vi "Growable Widget.vi"(8 "Error In":errorcluster, 10 "Widget Builder":refnum<class "Abstract Widget Builder.lvclass">) -> (0 "Error Out":errorcluster, 3 "New Growable Widget":refnum<class "Growable Widget.lvclass">)   [LabVIEW 2014, in "Dynamic GUI Composition and Management.lvlib" / "Growable Widget.lvclass"]
doc: "Copyright (c) 2016 Sze Howe Koh\nThis code is licensed under the MIT license"
uses:
  Growable Widget.lvclass
  Widget Builders/Abstract Widget Builder/Abstract Widget Builder.lvclass
  src/LabVIEW/Qt Widgets/QBoxLayout/Direction.ctl
  src/LabVIEW/Qt Widgets/QFrame/Shadow.ctl
  src/LabVIEW/Qt Widgets/QFrame/Shape.ctl
  Growable Widget.lvclass/Growable Widget.ctl
  src/LabVIEW/Qt Widgets/QFrame/setFrameShadow.vi
  src/LabVIEW/Qt Widgets/QFrame/setFrameShape.vi
  src/LabVIEW/LQ Core/LQCoreEngine/_Polymorphic Instances/Connect_CallbackIn_Void.vi
  src/LabVIEW/Qt Widgets/QComboBox/QComboBox.lvclass
  src/LabVIEW/Qt Widgets/QPushButton/QPushButton.lvclass
  src/LabVIEW/Qt Widgets/QBoxLayout/QBoxLayout.lvclass
  src/LabVIEW/Qt Widgets/QWidget/QWidget.lvclass
  src/LabVIEW/LQ Core/LQCoreEngine/LQCoreEngine.lvclass
  src/LabVIEW/Qt Widgets/QLineEdit/QLineEdit.lvclass
  src/LabVIEW/Qt Widgets/QFrame/QFrame.lvclass
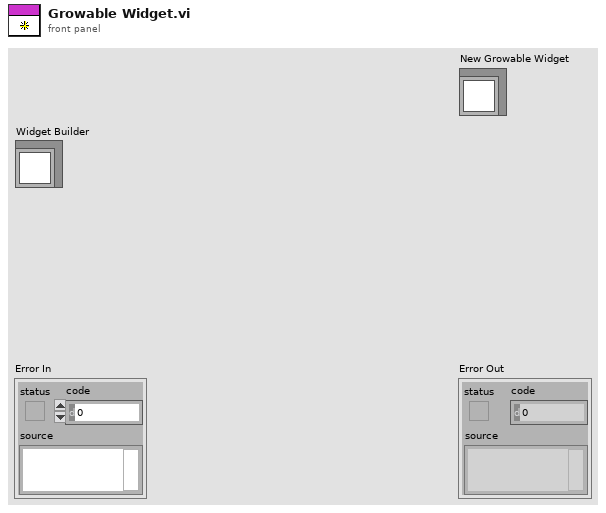
[diagram p1: front panel]
types:
  T1 = typedef "QFrame.lvclass/Shape.ctl" = i32
  T2 = typedef "QFrame.lvclass/Shadow.ctl" = i32
  T3 = typedef "QBoxLayout.lvclass/Direction.ctl" = i32
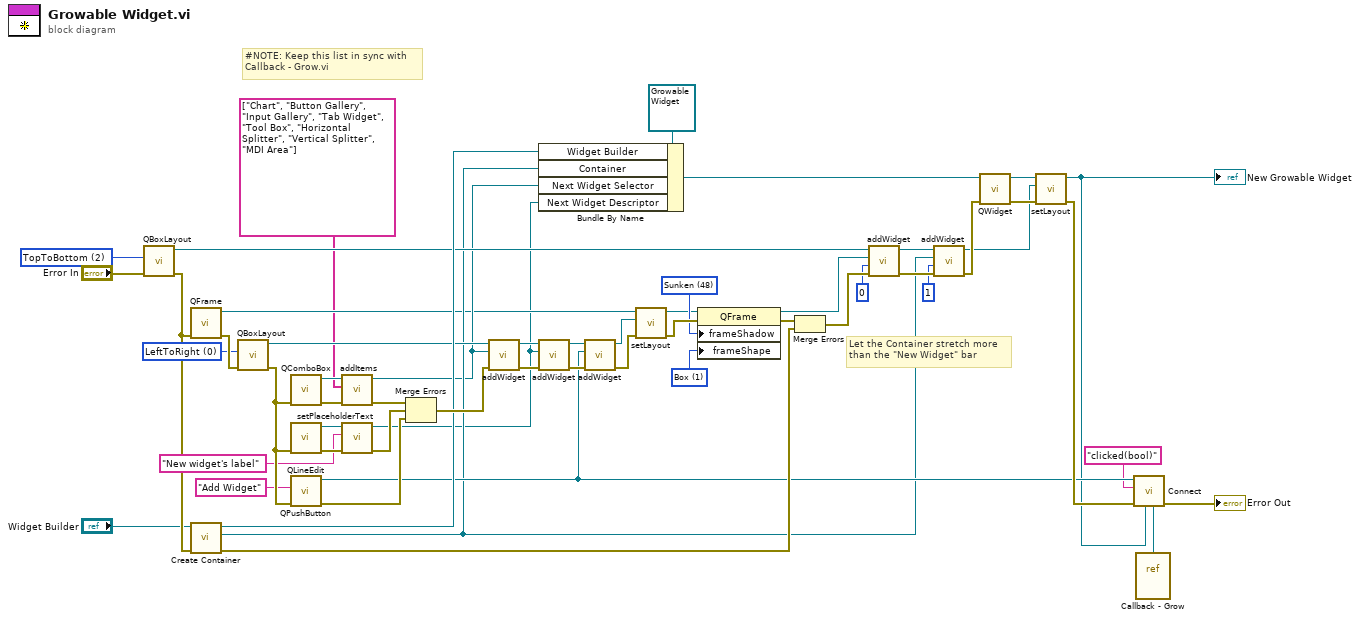
[diagram p0: block diagram]
diagram:
  w18 = T1 1 items=["NoFrame", "Box", "Panel", "HLine", "VLine", "StyledPanel"] ("frameShape")
  w19 = T2 48 items=["Plain"=16, "Raised"=32, "Sunken"=48] ("frameShadow")
  w36 = T3 2 items=["LeftToRight", "RightToLeft", "TopToBottom", "BottomToTop"] ("direction")
  w37 = T3 0 items=["LeftToRight", "RightToLeft", "TopToBottom", "BottomToTop"] ("direction")
  # "Let the Container stretch more\nthan the \"New Widget\" bar"
  # "#NOTE: Keep this list in sync with\nCallback - Grow.vi"
  n1 = call "QBoxLayout.vi"("Error In"="Error In", "direction"=w36) -> ("Error Out"=w54:errorcluster, "New QBoxLayout"=w32:refnum<class "QBoxLayout.lvclass">)  [unwired: 8 in]
  n2 = call "QFrame.vi"("Error In"=w54) -> ("Error Out"=w40:errorcluster, "New QFrame"=w20:refnum<class "QFrame.lvclass">)  [unwired: 9 in]
  n3 = call-dynamic "Create Container.vi"("Error In"=w54, "Abstract Widget Builder in"="Widget Builder") -> ("Error Out"=w53:errorcluster, "Container"=w24:refnum<class "QWidget.lvclass">, "Abstract Widget Builder out"=w48:refnum<class "Abstract Widget Builder.lvclass">)  [unwired: 7 in]
  n4 = call "QBoxLayout.vi"("Error In"=w40, "direction"=w37) -> ("Error Out"=w44:errorcluster, "New QBoxLayout"=w39:refnum<class "QBoxLayout.lvclass">)  [unwired: 8 in]
  n5 = call "QComboBox.vi"("Error In"=w44) -> ("Error Out"=w13:errorcluster, "New QComboBox"=w41:refnum<class "QComboBox.lvclass">)  [unwired: 9 in]
  n6 = call "QLineEdit.vi"("Error In"=w44) -> ("Error Out"=w4:errorcluster, "New QLineEdit"=w6:refnum<class "QLineEdit.lvclass">)  [unwired: 9 in]
  n7 = call "QPushButton.vi"("Error In"=w44, "text"="Add Widget") -> ("Error Out"=w43:errorcluster, "New QPushButton"=w26:refnum<class "QPushButton.lvclass">)  [unwired: 8 in]
  n8 = call "addItems.vi"("Error In"=w13, "texts"=string[] ["Chart", "Button Gallery", "Input Gallery", "Tab Widget", "Tool Box", "Horizontal Splitter", "Vertical Splitter", "MDI Area"], "QComboBox In"=w41) -> ("Error Out"=w12:errorcluster, "QComboBox Out"=w23:refnum<class "QComboBox.lvclass">)  [unwired: 7 in]
  n9 = call "setPlaceholderText.vi"("Error In"=w4, "text"="New widget's label", "QLineEdit In"=w6) -> ("Error Out"=w47:errorcluster, "QLineEdit Out"=w5:refnum<class "QLineEdit.lvclass">)  [unwired: 7 in]
  n10 = Merge Errors(w12, w47, w43) -> (w49:errorcluster)
  n11 = call "addWidget.vi"("Error In"=w49, "widget"=w23, "QBoxLayout In"=w39) -> ("Error Out"=w11:errorcluster, "QBoxLayout Out"=w22:refnum<class "QBoxLayout.lvclass">)  [unwired: 7 in]
  n12 = Bundle By Name(cluster=refnum<class "Growable Widget.lvclass"> refnum ("Growable Widget"), "Widget Builder"=w48, "Container"=w24, "Next Widget Selector"=w23, "Next Widget Descriptor"=w5) -> (w33:refnum<class "Growable Widget.lvclass">)
  n13 = call "addWidget.vi"("Error In"=w11, "widget"=w5, "QBoxLayout In"=w22) -> ("Error Out"=w46:errorcluster, "QBoxLayout Out"=w21:refnum<class "QBoxLayout.lvclass">)  [unwired: 7 in]
  n14 = call "addWidget.vi"("Error In"=w46, "widget"=w26, "QBoxLayout In"=w21) -> ("Error Out"=w10:errorcluster, "QBoxLayout Out"=w38:refnum<class "QBoxLayout.lvclass">)  [unwired: 7 in]
  n15 = call "setLayout.vi"("Error In"=w10, "layout"=w38, "QWidget In"=w20) -> ("Error Out"=w45:errorcluster, "QWidget Out"=w15:refnum<class "QFrame.lvclass">)  [unwired: 7 in]
  n16 = property class="QFrame"(reference=w15, error in=w45, "frameShadow"=w19, "frameShape"=w18) -> (reference out=w14:refnum<class "QFrame.lvclass">, error out=w2:errorcluster)
  n17 = Merge Errors(w2, w53) -> (w55:errorcluster)
  n18 = call "addWidget.vi"("Error In"=w55, "stretch"=0, "widget"=w14, "QBoxLayout In"=w32) -> ("Error Out"=w50:errorcluster, "QBoxLayout Out"=w31:refnum<class "QBoxLayout.lvclass">)  [unwired: 6 in]
  n19 = call "addWidget.vi"("Error In"=w50, "stretch"=1, "widget"=w24, "QBoxLayout In"=w31) -> ("Error Out"=w29:errorcluster, "QBoxLayout Out"=w28:refnum<class "QBoxLayout.lvclass">)  [unwired: 6 in]
  n20 = call "QWidget.vi"("Error In"=w29, "Post-Bundled Subclass"=w33) -> ("Error Out"=w51:errorcluster, "New QWidget"=w30:refnum<class "Growable Widget.lvclass">)  [unwired: 8 in]
  n21 = call "setLayout.vi"("Error In"=w51, "layout"=w28, "QWidget In"=w30) -> ("Error Out"=w52:errorcluster, "QWidget Out"=w25:refnum<class "Growable Widget.lvclass">)  [unwired: 7 in]
  "New Growable Widget" <- w25
  n22 = vi-ref "Callback - Grow.vi"() -> (w7:refnum<vi>)
  n23 = call-poly "Connect.vi"("Slot VI"=w7, "Receiver"=w25, "Error In"=w52, "Signal"="clicked(bool)", "Sender In"=w26) -> ("Error Out"=→"Error Out":errorcluster)  [unwired: 5 in, 1 out]
